vi "add_from_rio.vi"(4 "from_rio":cluster{"speed_is":dbl, "steering_is":dbl}, 5 "msg in":string) -> (2 "msg out":string)   [LabVIEW 2016]
uses:
  <userlib>/ROS for LabVIEW Software/ROS/MessageBuilding/std_msgs/subs/float64Scalar.vi
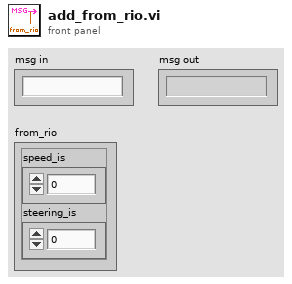
[diagram p1: front panel]
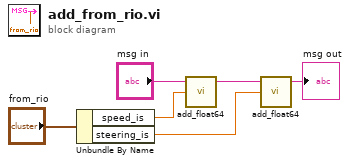
[diagram p0: block diagram]
diagram:
  n1 = Unbundle By Name("from_rio") -> ("speed_is"=w2:dbl, "steering_is"=w1:dbl)
  n2 = call-poly <userlib>:"add_float64.vi"("Numeric"=w2, "msg in"="msg in") -> ("msg out"=w4:string)  [unwired: 3 in]
  n3 = call-poly <userlib>:"add_float64.vi"("Numeric"=w1, "msg in"=w4) -> ("msg out"=→"msg out":string)  [unwired: 3 in]
